vi "Collect_data.vi"(1 "String":string, 2 "File Path":path) -> (0 "all rows":string[][](array[string]))   [LabVIEW 2025]
uses:
  <vilib>/Utility/file.llb/Read Delimited Spreadsheet (string).vi
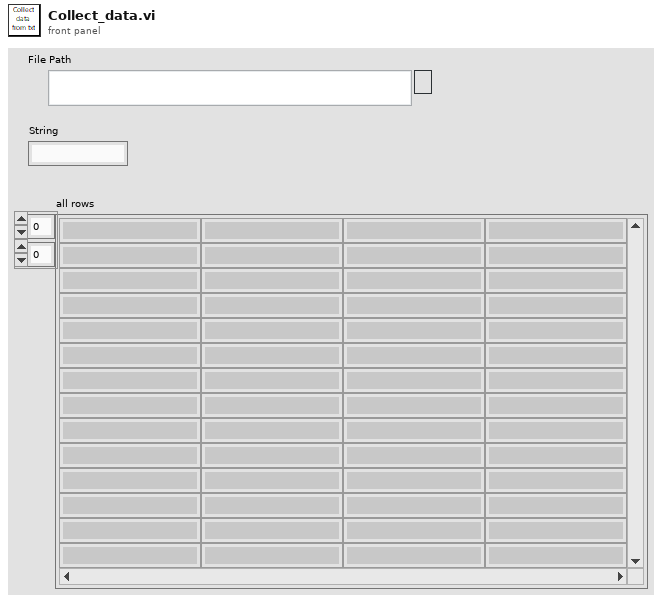
[diagram p1: front panel]
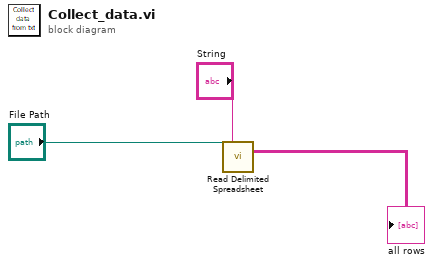
[diagram p0: block diagram]
diagram:
  n1 = call-poly <vilib>:"Read Delimited Spreadsheet.vi"("file path (dialog if empty)"="File Path", "format (%s)"="String") -> ("all rows"=→"all rows":string[][])  [unwired: 8 in, 5 out]
